vi "7-19-19 increasing.vi"() -> ()   [LabVIEW 2016]
uses:
  <userlib>/Levylab/LV to ITX/LVtoITX.lvclass
  <vilib>/Analysis/NI_AALPro.lvlib
panel:
  out "dG/dt Vs Temp Normalized vs prev":cluster{"Data":dbl[], "Data":dbl[]}[](graph)
  out "dG/dt Vs Temp Normalized vs 275K":cluster{"Data":dbl[], "Data":dbl[]}[](graph)
  out "dG/dt Vs Temp":cluster{"Data":dbl[], "Data":dbl[]}[](graph)
  out "output cluster":cluster{dbl[], dbl[], dbl[], dbl[]}
  out "G2T Vs Temp":cluster{"Data":dbl[], "Data":dbl[]}[](graph)
  out "Data":dbl[][](array[numeric])
  out "G Vs Time":cluster{"Data":dbl[], "Data":dbl[]}[](graph)
  out "Wavenames":string[](array[string])
  in  "Path":path=path "G:/My Drive/Data/SA40060.20190715.000000.dat"
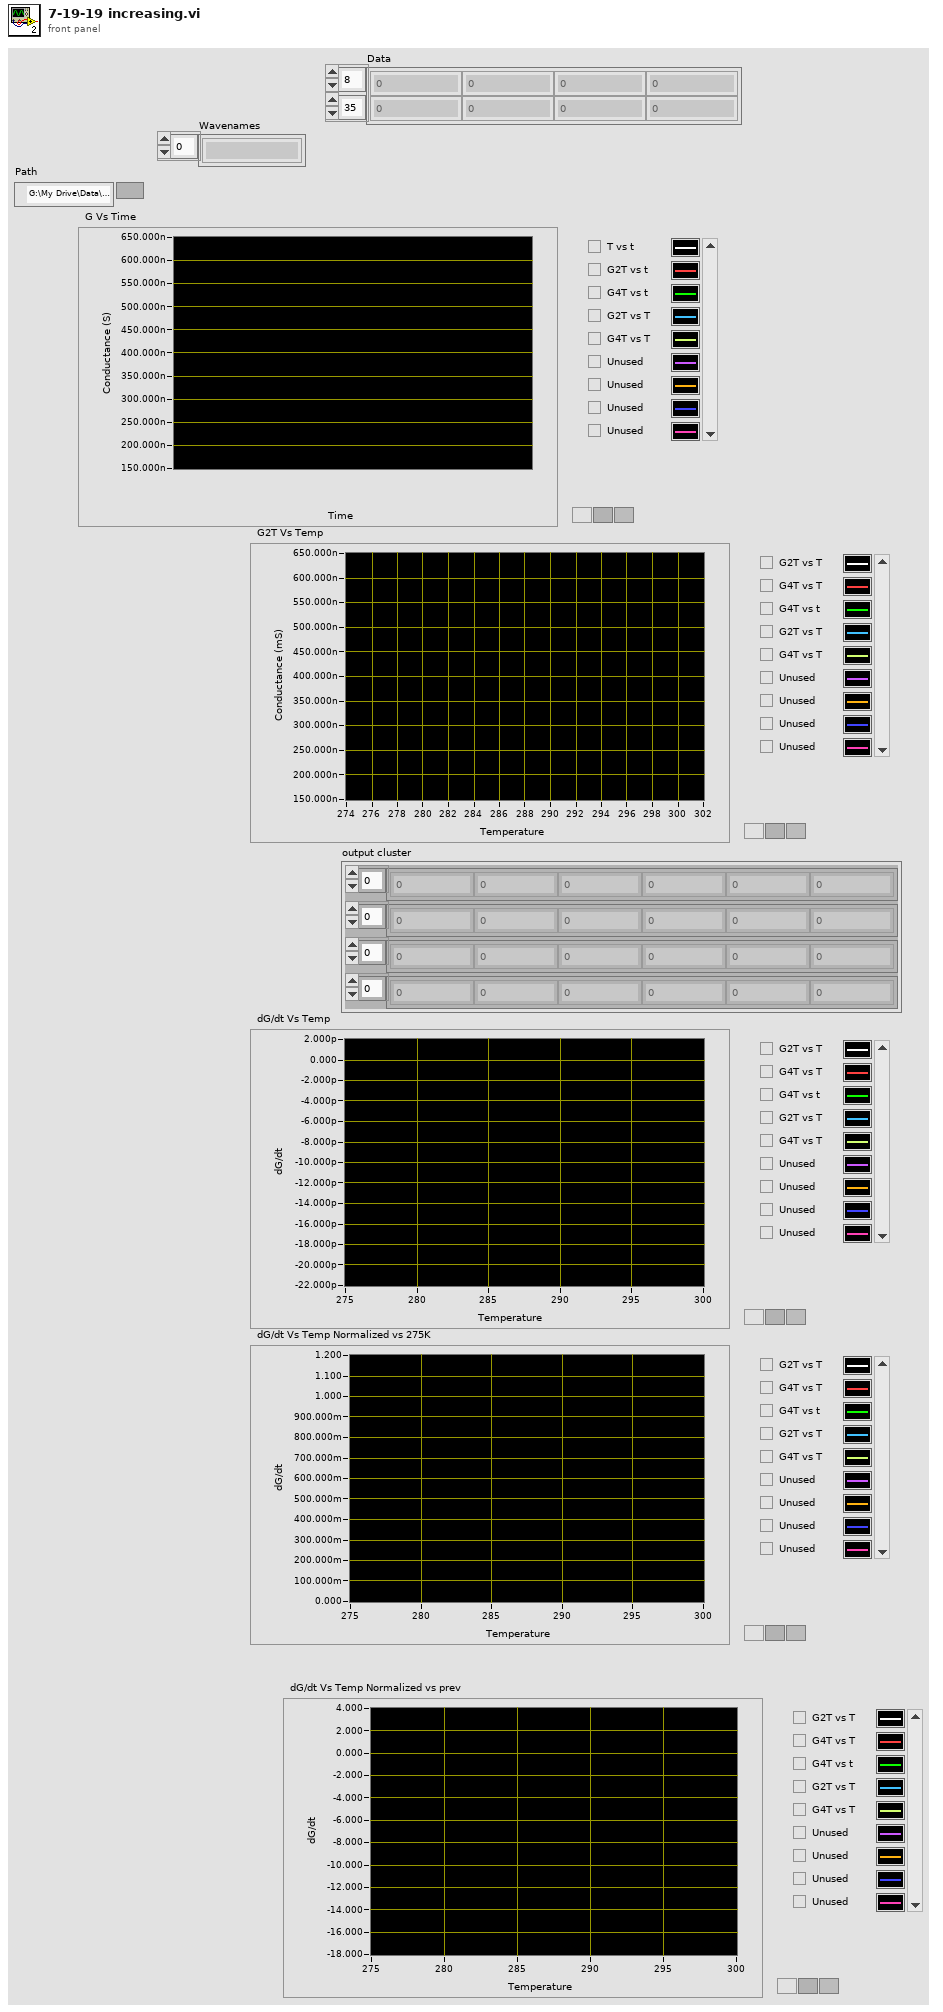
[diagram p1: front panel]
types:
  T1 = cluster{"slope min":dbl, "slope max":dbl, "intercept min":dbl, "intercept max":dbl}
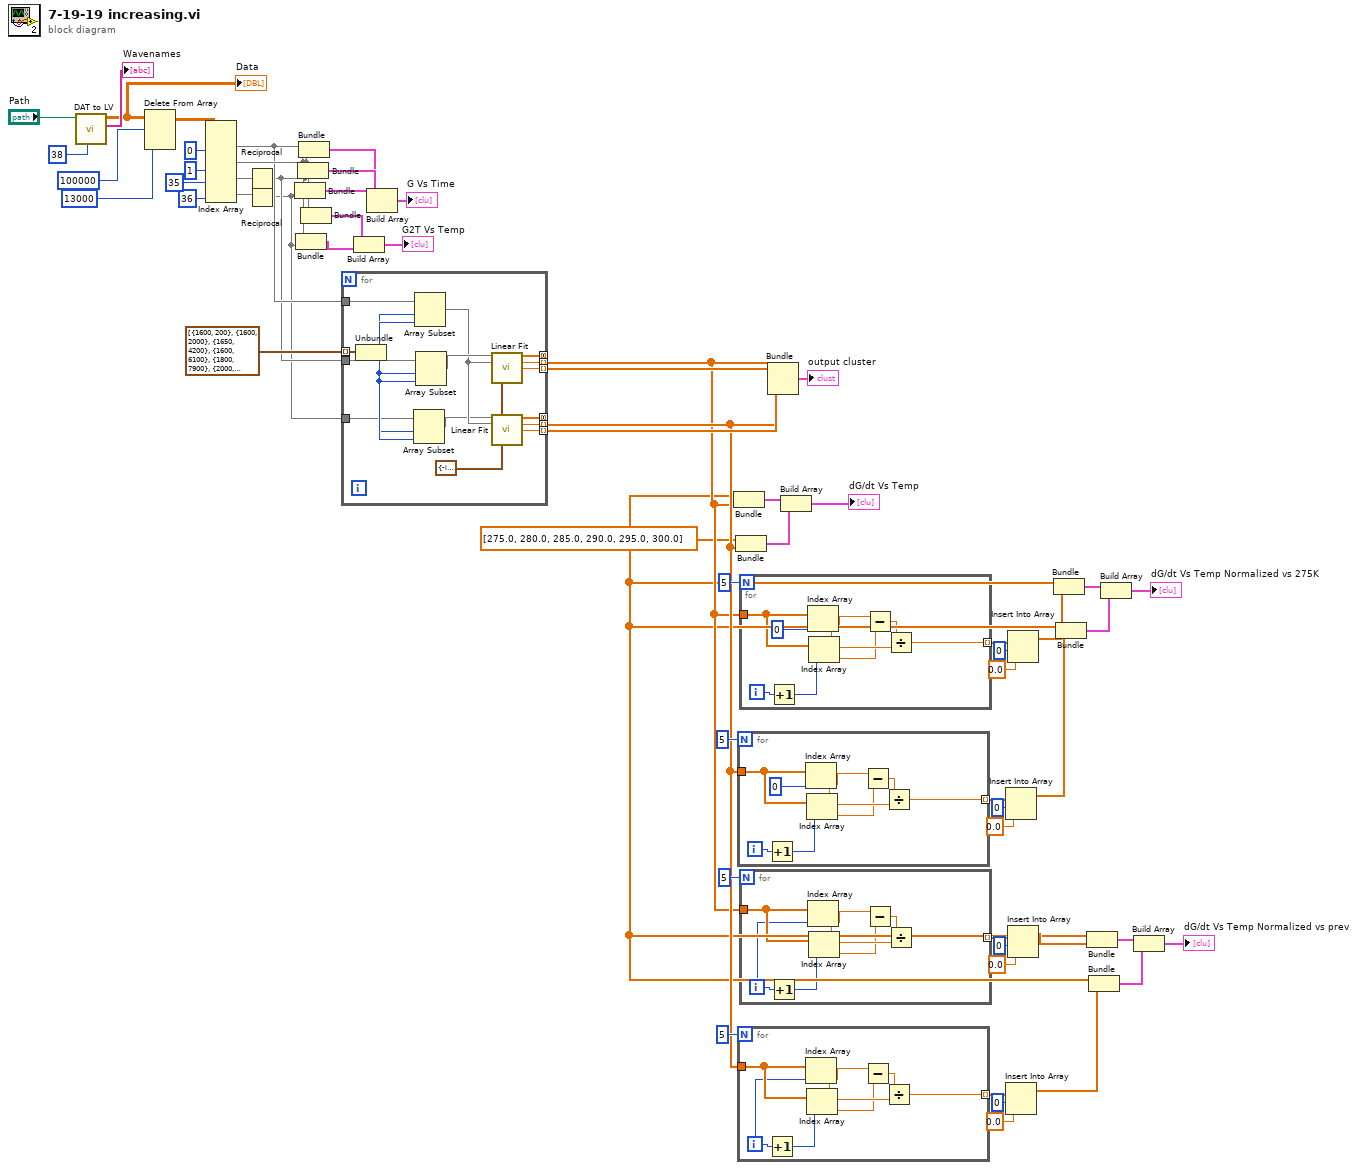
[diagram p0: block diagram]
diagram:
  w1 = dbl[] [275.0, 280.0, 285.0, 290.0, 295.0, 300.0]
  n1 = call <userlib>:"DAT to LV.vi"("header length"=38, "File Path"="Path") -> ("Wavenames"=→"Wavenames":string[], "Data"=w41:dbl[][])  [unwired: 6 in, 2 out]
  "Data" <- w41
  n2 = Delete From Array(array=w41, length=100000, index (row)=13000 ("index")) -> (array with subset deleted=w40:dbl[][])  [unwired: 1 in, 1 out]
  n3 = Index Array(array=w40, index (col) #1=0 ("disabled index (col)"), index (col) #2=1 ("index (col)"), index (col) #3=35 ("index (col)"), index (col) #4=36 ("index (col)")) -> (element #1=w38:dbl[], element #2=w53:dbl[], element #3=w48:dbl[], element #4=w47:dbl[])  [unwired: 4 in]
  n4 = Reciprocal(x=w48) -> (1/x=w37:dbl[])
  n5 = Reciprocal(x=w47) -> (1/x=w36:dbl[])
  n6 = Bundle("Data"=w38, w36) -> (w52:cluster{"Data":dbl[], dbl[]})  [unwired: 1 in]
  n7 = Bundle("Data"=w53, w36) -> (w45:cluster{"Data":dbl[], dbl[]})  [unwired: 1 in]
  n8 = Bundle("Data"=w38, w37) -> (w51:cluster{"Data":dbl[], dbl[]})  [unwired: 1 in]
  n9 = Bundle("Data"=w38, "Data"=w53) -> (w50:cluster{"Data":dbl[], "Data":dbl[]})  [unwired: 1 in]
  n10 = Bundle("Data"=w53, w37) -> (w46:cluster{"Data":dbl[], dbl[]})  [unwired: 1 in]
  n11 = for {
    tunnel: cluster{"length":i32, "index":i32}[] [{"length"=1600, "index"=200}, {"length"=1600, "index"=2000}, {"length"=1650, "index"=4200}, {"length"=1600, "index"=6100}, {"length"=1800, "index"=7900}, {"length"=2000, "index"=10000}] -> [w76] mode=indexing
    tunnel: w38 -> [w73]
    tunnel: w37 -> [w72]
    tunnel: w36 -> [w71]
    tunnel: [w66] -> _ mode=concatenating
    tunnel: [w65] -> _ mode=concatenating
    tunnel: [w64] -> w8 mode=indexing
    tunnel: [w63] -> w35 mode=indexing
    tunnel: [w62] -> w7 mode=indexing
    tunnel: [w61] -> w33 mode=indexing
    w67 = T1 {"slope min"=-inf, "slope max"=inf, "intercept min"=-inf, "intercept max"=inf} ("parameter bounds")
    n12 = Unbundle(w76) -> ("length"=w75:i32, "index"=w74:i32)
    n13 = Array Subset(array=w71, index=w74, length=w75) -> (w68:dbl[])
    n14 = Array Subset(array=w73, index=w74, length=w75) -> (w69:dbl[])
    n15 = Array Subset(array=w72, index=w74, length=w75) -> (w70:dbl[])
    n16 = call <vilib>:"Linear Fit.vi"("Y"=w70, "X"=w69, "parameter bounds"=w67) -> ("Best Linear Fit"=w66:dbl[], "slope"=w62:dbl, "intercept"=w61:dbl)  [unwired: 8 in, 2 out]
    n17 = call <vilib>:"Linear Fit.vi"("Y"=w68, "X"=w69, "parameter bounds"=w67) -> ("Best Linear Fit"=w65:dbl[], "slope"=w64:dbl, "intercept"=w63:dbl)  [unwired: 8 in, 2 out]
  }
  n18 = Build Array(w46, w45) -> (→"G2T Vs Temp":cluster{"Data":dbl[], dbl[]}[])
  n19 = Build Array(w50, w51, w52) -> (→"G Vs Time":cluster{"Data":dbl[], "Data":dbl[]}[])
  n20 = Bundle(w1, w7) -> (w31:cluster{dbl[], dbl[]})  [unwired: 1 in]
  n21 = Bundle(w1, w8) -> (w32:cluster{dbl[], dbl[]})  [unwired: 1 in]
  n22 = for {
    N: 5 -> [_]
    tunnel: w8 -> [w84]
    tunnel: [w77] -> w21 mode=indexing
    i -> [w82]
    n23 = Increment(x=w82) -> (x+1=w81:i32)
    n24 = Index Array(array=w84, index=0) -> (element=w79:dbl)
    n25 = Index Array(array=w84, index=w81) -> (element=w78:dbl)
    n26 = Subtract(x=w79, y=w78) -> (x-y=w80:dbl)
    n27 = Divide(x=w80, y=w79) -> (x/y=w77:dbl)
  }
  n28 = for {
    N: 5 -> [_]
    tunnel: w8 -> [w91]
    tunnel: [w86] -> w15 mode=indexing
    i -> [w85]
    n29 = Increment(x=w85) -> (x+1=w90:i32)
    n30 = Index Array(array=w91, index=w85) -> (element=w88:dbl)
    n31 = Index Array(array=w91, index=w90) -> (element=w87:dbl)
    n32 = Subtract(x=w88, y=w87) -> (x-y=w89:dbl)
    n33 = Divide(x=w89, y=w88) -> (x/y=w86:dbl)
  }
  n34 = for {
    N: 5 -> [_]
    tunnel: w7 -> [w99]
    tunnel: [w92] -> w28 mode=indexing
    i -> [w97]
    n35 = Increment(x=w97) -> (x+1=w96:i32)
    n36 = Index Array(array=w99, index=0) -> (element=w94:dbl)
    n37 = Index Array(array=w99, index=w96) -> (element=w93:dbl)
    n38 = Subtract(x=w94, y=w93) -> (x-y=w95:dbl)
    n39 = Divide(x=w95, y=w94) -> (x/y=w92:dbl)
  }
  n40 = for {
    N: 5 -> [_]
    tunnel: w7 -> [w106]
    tunnel: [w101] -> w10 mode=indexing
    i -> [w100]
    n41 = Increment(x=w100) -> (x+1=w105:i32)
    n42 = Index Array(array=w106, index=w100) -> (element=w103:dbl)
    n43 = Index Array(array=w106, index=w105) -> (element=w102:dbl)
    n44 = Subtract(x=w103, y=w102) -> (x-y=w104:dbl)
    n45 = Divide(x=w104, y=w103) -> (x/y=w101:dbl)
  }
  n46 = Bundle(w7, w33, w8, w35) -> (→"output cluster":cluster{dbl[], dbl[], dbl[], dbl[]})  [unwired: 1 in]
  n47 = Build Array(w31, w32) -> (→"dG/dt Vs Temp":cluster{dbl[], dbl[]}[])
  n48 = Insert Into Array(array=w21, index=0, new element=0.0 ("new element/subarray")) -> (w19:dbl[])
  n49 = Insert Into Array(array=w15, index=0, new element=0.0 ("new element/subarray")) -> (w3:dbl[])
  n50 = Insert Into Array(array=w28, index=0, new element=0.0 ("new element/subarray")) -> (w18:dbl[])
  n51 = Insert Into Array(array=w10, index=0, new element=0.0 ("new element/subarray")) -> (w2:dbl[])
  n52 = Bundle(w1, w18) -> (w25:cluster{dbl[], dbl[]})  [unwired: 1 in]
  n53 = Bundle(w1, w19) -> (w24:cluster{dbl[], dbl[]})  [unwired: 1 in]
  n54 = Bundle(w1, w2) -> (w4:cluster{dbl[], dbl[]})  [unwired: 1 in]
  n55 = Bundle(w1, w3) -> (w5:cluster{dbl[], dbl[]})  [unwired: 1 in]
  n56 = Build Array(w25, w24) -> (→"dG/dt Vs Temp Normalized vs 275K":cluster{dbl[], dbl[]}[])
  n57 = Build Array(w4, w5) -> (→"dG/dt Vs Temp Normalized vs prev":cluster{dbl[], dbl[]}[])
